vi "[GV]_Encoder Speed.vi"() -> ()   [LabVIEW 2016]
panel:
  in  "Encoder Speed":dbl
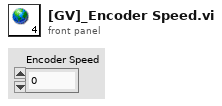
[diagram p1: front panel]
diagram:
